vi "UART Set.vi"(8 "error in (no error)":errorcluster, 11 "Command":string) -> (0 "error out":errorcluster)   [LabVIEW 2012]
uses:
  Libraries/uart_library.dll
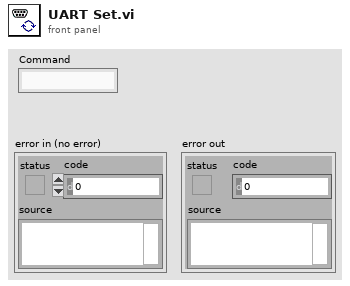
[diagram p1: front panel]
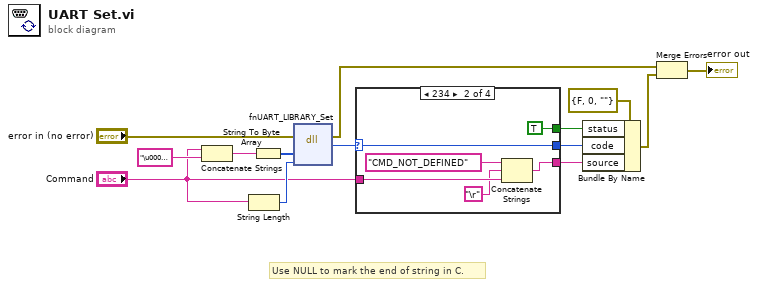
[diagram p0: block diagram]
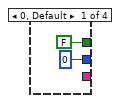
[diagram p2: hidden frame]
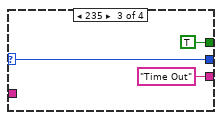
[diagram p3: hidden frame]
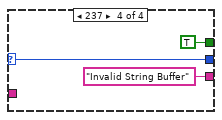
[diagram p4: hidden frame]
diagram:
  # "Use NULL to mark the end of string in C."
  n1 = Concatenate Strings("Command", "\u0000\u0000") -> (w3:string)
  n2 = String Length(string="Command") -> (length=w2:i32)
  n3 = String To Byte Array(string=w3) -> (unsigned byte array=w13:u8[])
  n4 = dll-call lib="C:/Leventhal lab VIs/Optogenetics/library-FilterWheel/Libraries/uart_library.dll" fn="fnUART_LIBRARY_Set"(error in="error in (no error)", "Command"=w13, "Length"=w2) -> (error out=w6:errorcluster, "return type"=w12:i32)  [unwired: 4 in, 1 out]
  n5 = case shown="234" w12 {
    selector: w12 -> [_ w21 w23 w26]
    tunnel: [_ w20 "Time Out" "Invalid String Buffer"] -> w7
    tunnel: [FALSE TRUE TRUE TRUE] -> w9
    tunnel: [0 w21 w23 w26] -> w8
    tunnel: "Command" -> [_ w18 _ _]
    frame 0, Default {
    }
    frame 234 {
      n6 = Concatenate Strings("CMD_NOT_DEFINED", "\r", w18) -> (w20:string)
    }
    frame 235 {
    }
    frame 237 {
    }
  }
  n7 = Bundle By Name(cluster=errorcluster {"status"=FALSE, "code"=0, "source"=""} ("error out"), "status"=w9, "code"=w8, "source"=w7) -> (w5:errorcluster)
  n8 = Merge Errors(w6, w5) -> (→"error out":errorcluster)
